vi "pH电极校准.vi"() -> ()   [LabVIEW 2016, in "斯坦道多参数.lvlib"]
uses:
  <vilib>/Utility/miscctls.llb/LVPointTypeDef.ctl
  <vilib>/Analysis/NI_AALBase.lvlib
panel:
  in  "校准停止":bool
  in  "校准启动":bool
  out "第二点校准值":dbl
  out "第一点校准值":dbl
  out "提示":string
  in  "校准模式":enum16{"两点校准", "单点校准"}(ring)
  out "最小值":sgl format="%#.2f"
  out "最大值":sgl format="%#.2f"
  out "变异系数":dbl format="%#.6f"
  out "standard deviation":dbl caption="标准差" format="%#.2f"
  out "mean":dbl caption="均值" format="%#.2f"
  out "波形图表":sgl(graph) caption="历史曲线"
  out "当前检测值":dbl format="%#.2g"
  out "标液2":dbl
  out "标液1":dbl
  out "当前信号值":dbl format="%#.2g"
  out "偏移值补偿":dbl format="%#.2g"
  out "电极斜率":dbl
  out "电极零点":dbl
  # "酸碱度电极设定"
  # "mV"
  # "mV"
  # "%"
  # "pH"
  # "请选择校准模式:"
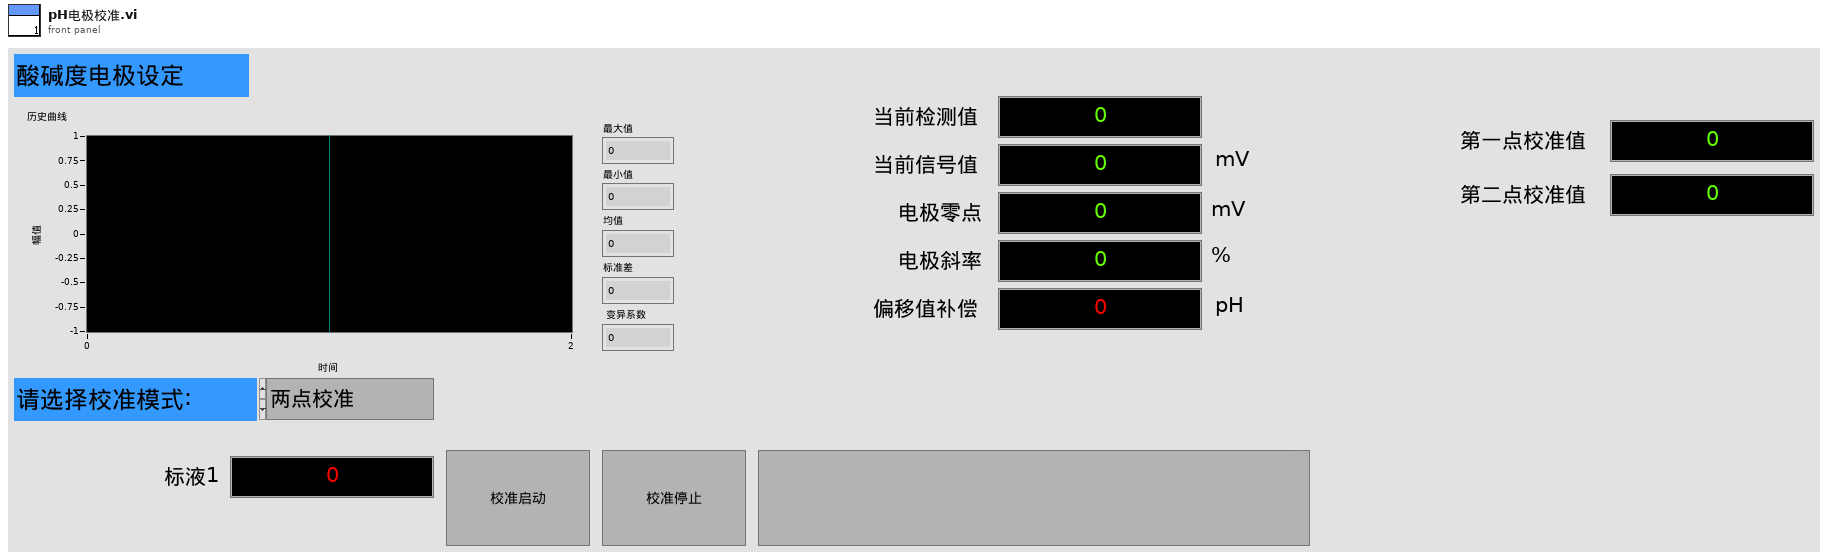
[diagram p1: front panel]
types:
  T1 = typedef "LVPointTypeDef.ctl" = cluster{"Horizontal":i16, "Vertical":i16}
  T2 = typedef "斯坦道多参数.lvlib/校准步骤.ctl" = enum16{"待机", "放置第一点标液", "第一点校准启动", "第一点校准写入", "第一点校准失败", "放置第二点标液", "第二点校准启动", "第二点校准写入", "第二点校准失败", "校准结果写入", "校准结束"}
  T3 = cluster{"电极状态标志":u16, "电极型号标志":u16, "酸碱度测量值":sgl, "温度测量值":sgl, "酸碱度信号值":sgl, "温度信号值":sgl, "酸碱度偏移修正值":sgl, "温度偏移修正值":sgl, "手动温度补偿值":sgl, "酸碱度电极零点":sgl, "酸碱度电极斜率":sgl, "第1点标准值记录":sgl, "第1点信号值记录":sgl, "第1点温度值记录":sgl, "第2点标准值记录":sgl, "第2点信号值记录":sgl, "第2点温度值记录":sgl, "命令滤波设定":u16, "温度模式":enum16{"ATC", "MTC"}, "生产批次":u16, "电极序号":u16, "串口地址":u16, "串口波特率":enum16{"9600", "19200", "115200"}, "串口校验位":enum16{"NONE", "ODD", "EVEN"}, "串口停止位":enum16{"1bit", "2bit"}, "第一点标准值":sgl, "第二点标准值":sgl}
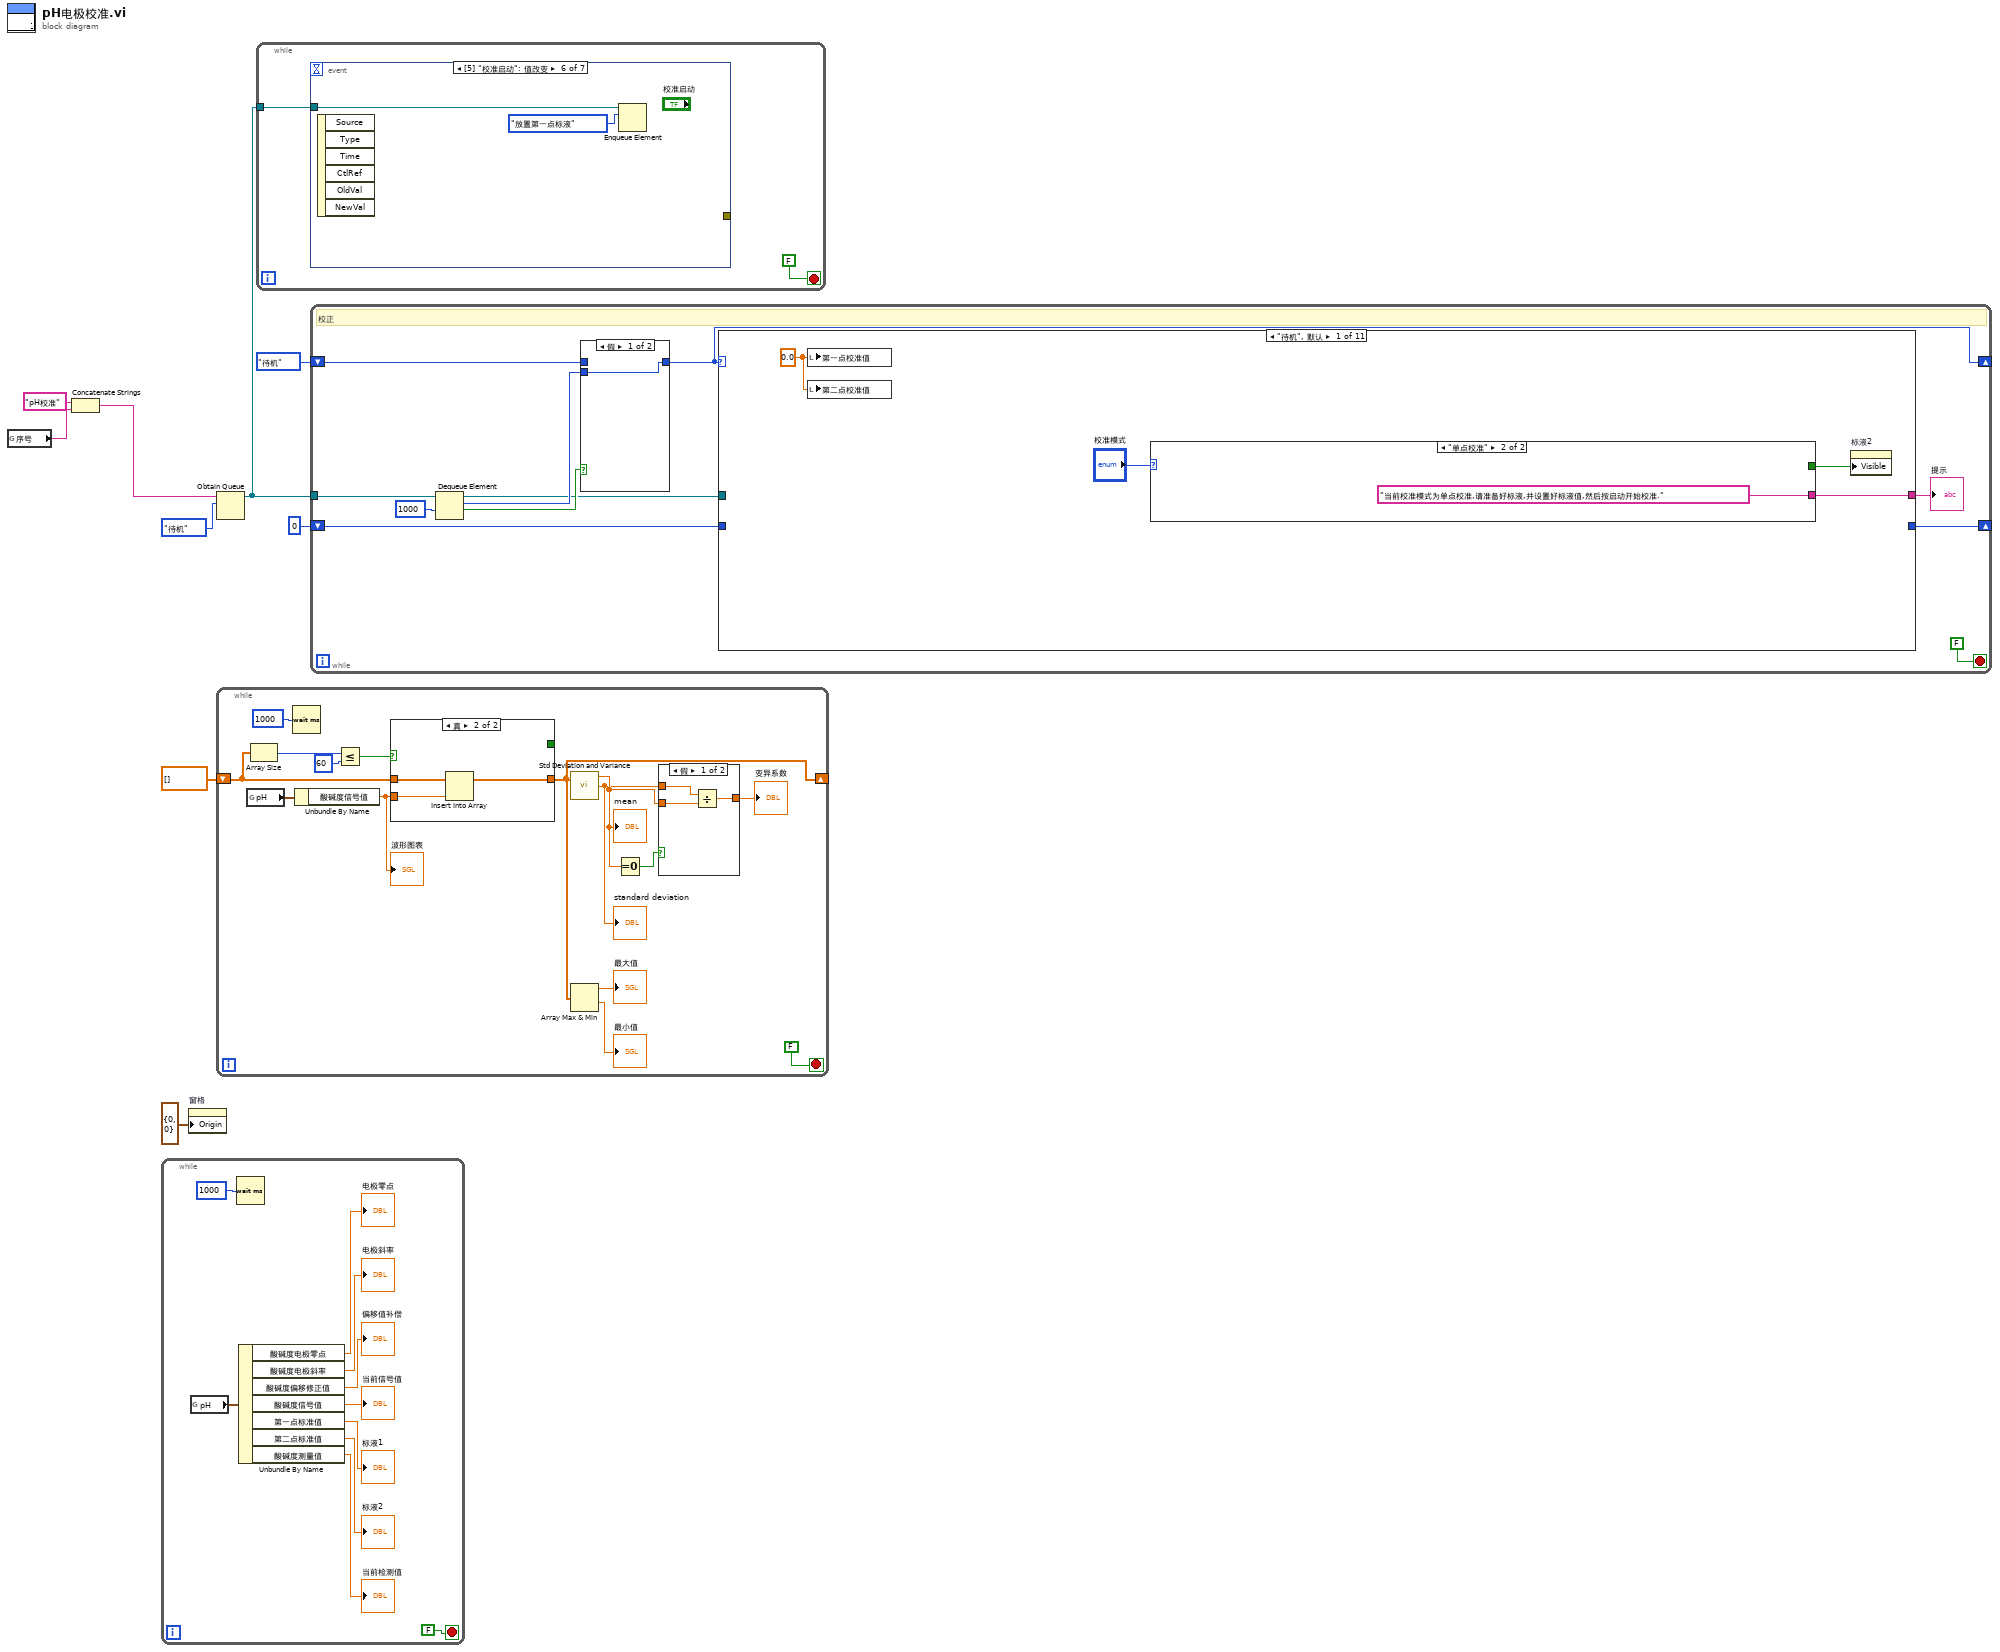
[diagram p0: block diagram]
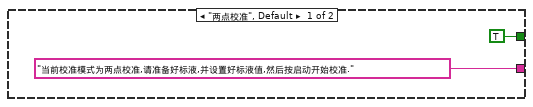
[diagram p3: hidden frame]
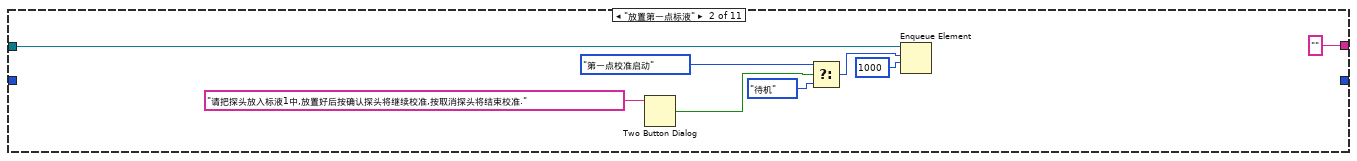
[diagram p4: hidden frame]
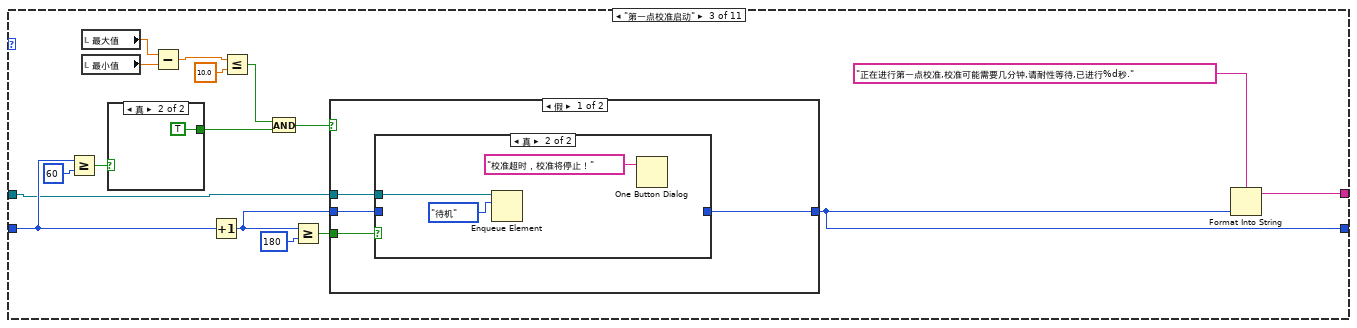
[diagram p5: hidden frame]
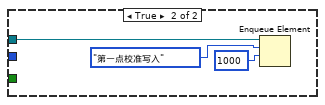
[diagram p7: hidden frame]
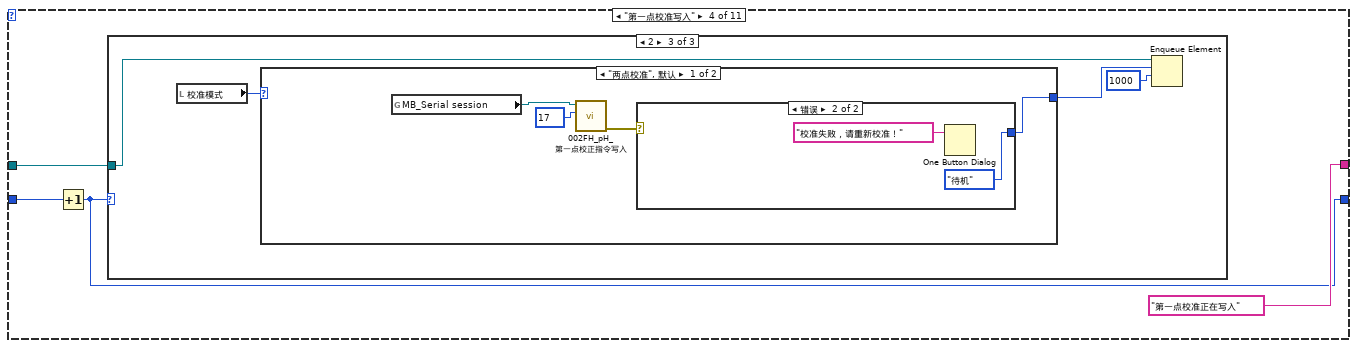
[diagram p9: hidden frame]
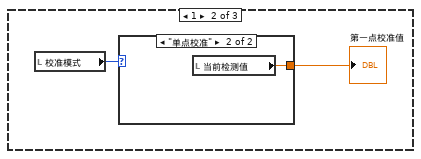
[diagram p11: hidden frame]
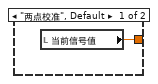
[diagram p12: hidden frame]
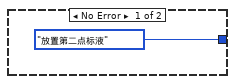
[diagram p13: hidden frame]
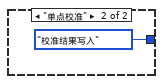
[diagram p14: hidden frame]
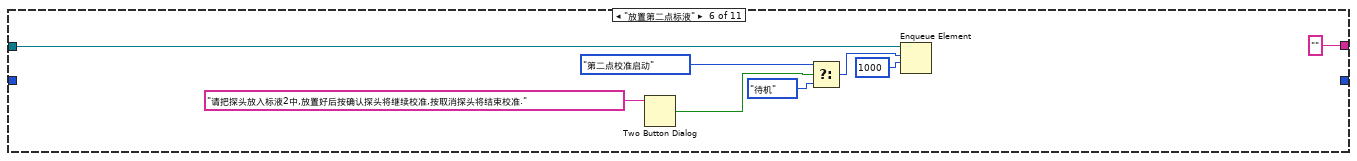
[diagram p16: hidden frame]
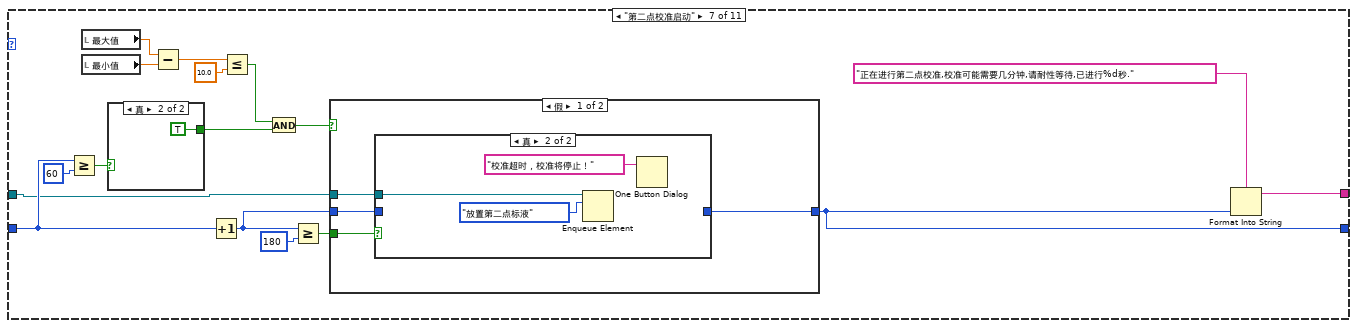
[diagram p17: hidden frame]
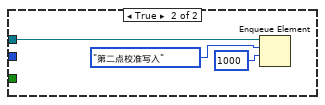
[diagram p19: hidden frame]
diagram:
  n1 = global read "多参数全局变量.vi" "序号"() -> (w1:string)
  n2 = Concatenate Strings("pH校准" ("名称（未命名）"), w1) -> (w2:string)
  n3 = while {
    stop <- FALSE stop-if-true
    n4 = global read "国弘过程全局变量.vi" "pH"() -> (w17:T3)
    n5 = Wait (ms)(milliseconds to wait=u32 1000 ("等待时间（毫秒）")) -> ()  [unwired: 1 out]
    n6 = Unbundle By Name(w17) -> ("酸碱度电极零点"=→"电极零点":sgl, "酸碱度电极斜率"=→"电极斜率":sgl, "酸碱度偏移修正值"=→"偏移值补偿":sgl, "酸碱度信号值"=→"当前信号值":sgl, "第一点标准值"=→"标液1":sgl, "第二点标准值"=→"标液2":sgl, "酸碱度测量值"=→"当前检测值":sgl)
  }
  n7 = property on="窗格" class="Pane"("Origin"=T1 {"Horizontal"=0, "Vertical"=0} ("原点")) -> ()  [unwired: 2 in, 2 out]
  n8 = Obtain Queue(name (unnamed)=w2, element data type=校准步骤."待机" ("枚举")) -> (queue out=w4:refnum<queue>)  [unwired: 3 in, 2 out]
  n9 = while {
    shift-right: [w26] -> _
    shift-left: sgl[] [] -> [w30]
    stop <- FALSE stop-if-true
    n10 = global read "国弘过程全局变量.vi" "pH"() -> (w27:T3)
    n11 = Array Size(array=w30) -> (size(s)=w32:i32)
    n12 = Wait (ms)(milliseconds to wait=u32 1000 ("等待时间（毫秒）")) -> ()  [unwired: 1 out]
    n13 = Unbundle By Name(w27) -> ("酸碱度信号值"=w20:sgl)
    "波形图表" <- w20
    n14 = Less Or Equal?(x=w32, y=60) -> (x <= y?=w31:bool)
    n15 = case shown="真" w31 {
      tunnel: w30 -> [w43 w46]
      tunnel: w20 -> [w41 w45]
      tunnel: [w39 w44] -> w26
      tunnel: [TRUE _] -> _
      frame False {
        n16 = Replace Array Subset(array=w43, new element=w41) -> (w42:sgl[])  [unwired: 1 in]
        n17 = Rotate 1D Array(1:w42, 2:-1 ("n")) -> (0:w39:sgl[])
      }
      frame True {
        n18 = Insert Into Array(array=w46, new element=w45) -> (w44:sgl[])  [unwired: 1 in]
      }
    }
    n19 = call <vilib>:"Std Deviation and Variance.vi"("X"=w26) -> ("mean"=w22:dbl, "standard deviation"=w21:dbl)  [unwired: 1 in, 1 out]
    "mean" <- w22
    "standard deviation" <- w21
    n20 = Array Max & Min(array=w26) -> (max value=→"最大值":sgl, min value=→"最小值":sgl)  [unwired: 2 out]
    n21 = Equal To 0?(x=w22) -> (x = 0?=w29:bool)
    n22 = case shown="假" w29 {
      tunnel: w21 -> [w37 _]
      tunnel: [w36 _] -> w23
      tunnel: w22 -> [w35 _]
      frame False {
        n23 = Divide(x=w37, y=w35) -> (x/y=w36:dbl)
      }
      frame True {
      }
    }
    "变异系数" <- w23
  }
  n24 = while {
    tunnel: w4 -> [w47]
    stop <- FALSE stop-if-true
    n25 = event shown="[5] \"校准启动\": 值改变" {
      selector: _ -> [_ _ _ _ _ _ _]
      dyn-events: _ -> [_ _ _ _ _ _ _]
      timeout: _ -> [_ _ _ _ _ _ _]
      tunnel: [_ _ w54 w57 w60 _ _] -> _
      tunnel: w47 -> [_ _ _ _ _ w62 w64]
      event Timeout {
        n26 = event-data() -> ()  [unwired: 1 in, 3 out]
      }
      event "标液1", "标液2", "偏移值补偿": Mouse Down {
        n27 = event-data() -> ("CtlRef"=w52:refnum<vi>)  [unwired: 1 in, 7 out]
        n28 = property class="DigNum (严格)"(reference=w52) -> (reference out=w49:refnum<vi>, "Value"=w50:dbl)  [unwired: 1 in, 1 out]
        n29 = call "数字键盘.vi"("OldNumber"=w50) -> ("NewNumber"=w51:sgl)
        n30 = property class="DigNum (严格)"(reference=w49, "Val(Sgnl)"=w51) -> ()  [unwired: 1 in, 2 out]
      }
      event "偏移值补偿": Value Change {
        n31 = event-data() -> ("NewVal"=w55:dbl)  [unwired: 1 in, 5 out]
        n32 = global read "多参数全局变量.vi" "MB_Serial session"() -> (w53:refnum<class "MB_Master_Serial.lvclass">)
        n33 = call "000CH_pH_pH偏移修正值写入.vi"("数值"=w55, "MB_Serial session in"=w53) -> ("error out"=w54:errorcluster)  [unwired: 8 in, 1 out]
      }
      event "标液1": Value Change {
        n34 = event-data() -> ("NewVal"=w58:dbl)  [unwired: 1 in, 5 out]
        n35 = global read "多参数全局变量.vi" "MB_Serial session"() -> (w56:refnum<class "MB_Master_Serial.lvclass">)
        n36 = call "0030H_pH_第一点标准值写入.vi"("数值"=w58, "MB_Serial session in"=w56) -> ("error out"=w57:errorcluster)  [unwired: 8 in, 1 out]
      }
      event "标液2": Value Change {
        n37 = event-data() -> ("NewVal"=w61:dbl)  [unwired: 1 in, 5 out]
        n38 = global read "多参数全局变量.vi" "MB_Serial session"() -> (w59:refnum<class "MB_Master_Serial.lvclass">)
        n39 = call "0033H_pH_第二点标准值写入.vi"("数值"=w61, "MB_Serial session in"=w59) -> ("error out"=w60:errorcluster)  [unwired: 8 in, 1 out]
      }
      event "校准启动": Value Change {
        n40 = event-data() -> ()  [unwired: 1 in, 6 out]
        n41 = Enqueue Element(queue=w62, element=校准步骤."放置第一点标液" ("元素")) -> ()  [unwired: 2 in, 3 out]
      }
      event "校准停止": Value Change {
        n42 = event-data() -> ()  [unwired: 1 in, 6 out]
        n43 = Flush Queue(queue=w64) -> (queue out=w65:refnum<queue>)  [unwired: 1 in, 2 out]
        n44 = Enqueue Element(queue=w65, element=校准步骤."待机" ("元素"), timeout in ms (-1)=1000 ("超时毫秒(-1)")) -> ()  [unwired: 1 in, 3 out]
      }
    }
  }
  n45 = while "While循环" {
    shift-right: [w69] -> _
    shift-left: 校准步骤."待机" ("枚举") -> [w70]
    shift-right: [w76] -> _
    shift-left: 0 -> [w77]
    tunnel: w4 -> [w74]
    stop <- FALSE stop-if-true
    # "校正"
    n46 = Dequeue Element(queue=w74, timeout in ms (-1)=1000 ("超时毫秒(-1)")) -> (queue out=w68:refnum<queue>, element=w71:T2, timed out?=w72:bool)  [unwired: 1 in, 1 out]
    n47 = case shown="假" w72 {
      tunnel: w71 -> [w79 _]
      tunnel: [w79 w80] -> w69
      tunnel: w70 -> [_ w80]
      frame False {
      }
      frame True {
      }
    }
    n48 = case shown="\"待机\", 默认" w69 {
      tunnel: [w84 "" ("提示") w111 "第一点校准正在写入" ("提示") _ "" ("提示") w168 "第二点校准正在写入" ("提示") _ w199 w227] -> w75
      tunnel: w77 -> [_ _ w105 w127 _ _ w162 w184 _ _ _]
      tunnel: [_ _ w96 w126 _ _ w153 w183 _ _ _] -> w76
      tunnel: w68 -> [_ w94 w99 w125 _ w151 w156 w182 _ w198 _]
      frame "待机", Default {
        w81 = 0.0 ("第一点校准值")
        n49 = local write "第一点校准值"(w81) -> ()
        n50 = local write "第二点校准值"(w81) -> ()
        n51 = case shown="\"单点校准\"" "校准模式" {
          tunnel: ["当前校准模式为两点校准,请准备好标液,并设置好标液值,然后按启动开始校准." ("提示") "当前校准模式为单点校准,请准备好标液,并设置好标液值,然后按启动开始校准." ("提示")] -> w84
          tunnel: [TRUE ("可见") _] -> w83
          frame "两点校准", Default {
          }
          frame "单点校准" {
          }
        }
        n52 = property on="标液2" class="DigNum (严格)"("Visible"=w83) -> ()  [unwired: 2 in, 2 out]
      }
      frame "放置第一点标液" {
        n53 = Two Button Dialog(message="请把探头放入标液1中,放置好后按确认探头将继续校准,按取消探头将结束校准." ("消息")) -> (T button?=w92:bool)  [unwired: 2 in]
        n54 = Select(t=校准步骤."第一点校准启动" ("元素"), s=w92, f=校准步骤."待机" ("元素")) -> (s? t:f=w89:T2)
        n55 = Enqueue Element(queue=w94, element=w89, timeout in ms (-1)=1000 ("超时毫秒(-1)")) -> ()  [unwired: 1 in, 3 out]
      }
      frame "第一点校准启动" {
        n56 = Greater Or Equal?(x=w105, y=60) -> (x >= y?=w106:bool)
        n57 = local read "最大值"() -> (w102:sgl)
        n58 = local read "最小值"() -> (w103:sgl)
        n59 = case shown="真" w106 {
          tunnel: [_ TRUE] -> w104
          frame False {
          }
          frame True {
          }
        }
        n60 = Subtract(x=w102, y=w103) -> (x-y=w101:sgl)
        n61 = Increment(x=w105) -> (x+1=w97:i32)
        n62 = Less Or Equal?(x=w101, y=10.0) -> (x <= y?=w109:bool)
        n63 = And(x=w109, y=w104) -> (x .and. y?=w100:bool)
        n64 = Greater Or Equal?(x=w97, y=180) -> (x >= y?=w98:bool)
        n65 = case shown="假" w100 {
          tunnel: w99 -> [w115 w123]
          tunnel: w98 -> [w116 _]
          tunnel: w97 -> [w114 _]
          tunnel: [w113 _] -> w96
          frame False {
            n66 = case shown="真" w116 {
              tunnel: w115 -> [_ w120]
              tunnel: w114 -> [w117 _]
              tunnel: [w117 _] -> w113
              frame False {
              }
              frame True {
                n67 = Enqueue Element(queue=w120, element=校准步骤."待机" ("元素")) -> ()  [unwired: 2 in, 3 out]
                n68 = One Button Dialog(message="校准超时，校准将停止！" ("消息")) -> ()  [unwired: 1 in, 1 out]
              }
            }
          }
          frame True {
            n69 = Enqueue Element(queue=w123, element=校准步骤."第一点校准写入" ("元素"), timeout in ms (-1)=1000 ("超时毫秒(-1)")) -> ()  [unwired: 1 in, 3 out]
          }
        }
        n70 = Format Into String(format string="正在进行第一点校准,校准可能需要几分钟,请耐性等待,已进行%d秒." ("格式字符串"), w96) -> (resulting string=w111:string)  [unwired: 2 in, 1 out]
      }
      frame "第一点校准写入" {
        n71 = Increment(x=w127) -> (x+1=w126:i32)
        n72 = case shown="2" w126 {
          tunnel: w125 -> [_ _ w136]
          frame 0, Default {
          }
          frame 1 {
            n73 = local read "校准模式"() -> (w129:enum16{"两点校准", "单点校准"})
            n74 = case shown="\"单点校准\"" w129 {
              tunnel: [w131 w132] -> w130
              frame "两点校准", Default {
                n75 = local read "当前信号值"() -> (w131:dbl)
              }
              frame "单点校准" {
                n76 = local read "当前检测值"() -> (w132:dbl)
              }
            }
            "第一点校准值" <- w130
          }
          frame 2 {
            n77 = local read "校准模式"() -> (w135:enum16{"两点校准", "单点校准"})
            n78 = case shown="\"两点校准\", 默认" w135 {
              tunnel: [w140 校准步骤."校准结果写入" ("元素")] -> w134
              frame "两点校准", Default {
                n79 = global read "多参数全局变量.vi" "MB_Serial session"() -> (w139:refnum<class "MB_Master_Serial.lvclass">)
                n80 = call "002FH_pH_第一点校正指令写入.vi"("数值"=u16 17, "MB_Serial session in"=w139) -> ("error out"=w137:errorcluster)  [unwired: 8 in, 1 out]
                n81 = case shown="错误" w137 {
                  tunnel: [校准步骤."放置第二点标液" ("元素") 校准步骤."待机" ("元素")] -> w140
                  frame No Error {
                  }
                  frame Error {
                    n82 = One Button Dialog(message="校准失败，请重新校准！" ("消息")) -> ()  [unwired: 1 in, 1 out]
                  }
                }
              }
              frame "单点校准" {
              }
            }
            n83 = Enqueue Element(queue=w136, element=w134, timeout in ms (-1)=1000 ("超时毫秒(-1)")) -> ()  [unwired: 1 in, 3 out]
          }
        }
      }
      frame "第一点校准失败" {
      }
      frame "放置第二点标液" {
        n84 = Two Button Dialog(message="请把探头放入标液2中,放置好后按确认探头将继续校准,按取消探头将结束校准." ("消息")) -> (T button?=w149:bool)  [unwired: 2 in]
        n85 = Select(t=校准步骤."第二点校准启动" ("元素"), s=w149, f=校准步骤."待机" ("元素")) -> (s? t:f=w146:T2)
        n86 = Enqueue Element(queue=w151, element=w146, timeout in ms (-1)=1000 ("超时毫秒(-1)")) -> ()  [unwired: 1 in, 3 out]
      }
      frame "第二点校准启动" {
        n87 = Greater Or Equal?(x=w162, y=60) -> (x >= y?=w163:bool)
        n88 = local read "最大值"() -> (w159:sgl)
        n89 = local read "最小值"() -> (w160:sgl)
        n90 = case shown="真" w163 {
          tunnel: [_ TRUE] -> w161
          frame False {
          }
          frame True {
          }
        }
        n91 = Subtract(x=w159, y=w160) -> (x-y=w158:sgl)
        n92 = Increment(x=w162) -> (x+1=w154:i32)
        n93 = Less Or Equal?(x=w158, y=10.0) -> (x <= y?=w166:bool)
        n94 = And(x=w166, y=w161) -> (x .and. y?=w157:bool)
        n95 = Greater Or Equal?(x=w154, y=180) -> (x >= y?=w155:bool)
        n96 = case shown="假" w157 {
          tunnel: w156 -> [w172 w180]
          tunnel: w155 -> [w173 _]
          tunnel: w154 -> [w171 _]
          tunnel: [w170 _] -> w153
          frame False {
            n97 = case shown="真" w173 {
              tunnel: w172 -> [_ w177]
              tunnel: w171 -> [w174 _]
              tunnel: [w174 _] -> w170
              frame False {
              }
              frame True {
                n98 = Enqueue Element(queue=w177, element=校准步骤."放置第二点标液" ("元素")) -> ()  [unwired: 2 in, 3 out]
                n99 = One Button Dialog(message="校准超时，校准将停止！" ("消息")) -> ()  [unwired: 1 in, 1 out]
              }
            }
          }
          frame True {
            n100 = Enqueue Element(queue=w180, element=校准步骤."第二点校准写入" ("元素"), timeout in ms (-1)=1000 ("超时毫秒(-1)")) -> ()  [unwired: 1 in, 3 out]
          }
        }
        n101 = Format Into String(format string="正在进行第二点校准,校准可能需要几分钟,请耐性等待,已进行%d秒." ("格式字符串"), w153) -> (resulting string=w168:string)  [unwired: 2 in, 1 out]
      }
      frame "第二点校准写入" {
        n102 = Increment(x=w184) -> (x+1=w183:i32)
        n103 = case shown="2" w183 {
          tunnel: w182 -> [_ _ w192]
          frame 0, Default {
          }
          frame 1 {
            n104 = local read "当前信号值"() -> (→"第二点校准值":dbl)
          }
          frame 2 {
            n105 = global read "多参数全局变量.vi" "MB_Serial session"() -> (w189:refnum<class "MB_Master_Serial.lvclass">)
            n106 = call "0032H_pH_第二点校正指令写入.vi"("数值"=u16 33, "MB_Serial session in"=w189) -> ("error out"=w188:errorcluster)  [unwired: 8 in, 1 out]
            n107 = case shown="错误" w188 {
              tunnel: [校准步骤."校准结果写入" ("元素") 校准步骤."放置第二点标液" ("元素")] -> w187
              frame No Error {
              }
              frame Error {
                n108 = One Button Dialog(message="校准失败，请重新校准！" ("消息")) -> ()  [unwired: 1 in, 1 out]
              }
            }
            n109 = Enqueue Element(queue=w192, element=w187, timeout in ms (-1)=1000 ("超时毫秒(-1)")) -> ()  [unwired: 1 in, 3 out]
          }
        }
      }
      frame "第二点校准失败" {
      }
      frame "校准结果写入" {
        n110 = Enqueue Element(queue=w198, element=校准步骤."校准结束" ("元素")) -> ()  [unwired: 2 in, 3 out]
        n111 = local read "校准模式"() -> (w196:enum16{"两点校准", "单点校准"})
        n112 = case shown="\"单点校准\"" w196 {
          tunnel: [w202 w221] -> w199
          frame "两点校准", Default {
            n113 = global read "国弘过程全局变量.vi" "pH"() -> (w201:T3)
            n114 = Unbundle By Name(w201) -> ("电极状态标志"=w200:u16)
            n115 = case shown="0, 默认" w200 {
              selector: w200 -> [w204 _ w213]
              tunnel: [w203 w208 w212] -> w202
              frame 0, Default {
                n116 = case shown="0, 默认" w204 {
                  tunnel: ["校正未正常启动，请重新校正" "第一点校准通过" "第二点校准通过"] -> w203
                  frame 0, Default {
                  }
                  frame 1 {
                  }
                  frame 2 {
                  }
                }
              }
              frame 2 {
                n117 = local read "第一点校准值"() -> (w210:dbl)
                n118 = local read "第二点校准值"() -> (w211:dbl)
                n119 = Format Into String(format string="两点校准结果：\n第一点校准值：%f\n第二点校准值：%f" ("提示"), w210, w211) -> (resulting string=w208:string)  [unwired: 2 in, 1 out]
              }
              frame 3, 4 {
                n120 = case shown="4" w213 {
                  tunnel: ["校正失败，电极零点超出范围" "校正失败，电极斜率超出范围"] -> w212
                  frame 3, Default {
                  }
                  frame 4 {
                  }
                }
              }
            }
          }
          frame "单点校准" {
            n121 = local read "当前检测值"() -> (w220:dbl)
            n122 = local read "标液1"() -> (w219:dbl)
            n123 = global read "多参数全局变量.vi" "MB_Serial session"() -> (w218:refnum<class "MB_Master_Serial.lvclass">)
            n124 = Subtract(x=w219, y=w220) -> (x-y=w216:dbl)
            n125 = call "000CH_pH_pH偏移修正值写入.vi"("数值"=w216, "MB_Serial session in"=w218) -> ("error out"=w217:errorcluster)  [unwired: 8 in, 1 out]
            n126 = case shown="无错误" w217 {
              tunnel: [w222 "校准失败"] -> w221
              frame No Error {
                n127 = local read "第一点校准值"() -> (w224:dbl)
                n128 = Format Into String(format string="单点校准结果：\n校准值：%f" ("提示"), w224) -> (resulting string=w222:string)  [unwired: 2 in, 1 out]
              }
              frame Error {
                n129 = One Button Dialog(message="校准失败，请重新校准！" ("消息")) -> ()  [unwired: 1 in, 1 out]
              }
            }
          }
        }
        n130 = One Button Dialog(message=w199) -> ()  [unwired: 1 in, 1 out]
      }
      frame "校准结束" {
        n131 = local read "提示"() -> (w227:string)
      }
    }
    "提示" <- w75
  }
